vi "Posture Rotation.vi"(10 "Rotation X,Y,Z":cluster{"X":dbl, "Y":dbl, "Z":dbl}) -> (0 "angles":cluster{"roll":dbl, "pitch":dbl, "yaw":dbl}, 1 "Rotation Vector":dbl[](array[numeric]), 2 "Rotation Angle":dbl, 3 "data out":T1)   [LabVIEW 2021]
doc: "This VI calculates the Rotation Angle and Rotation\nVector between gravity acceleration in myRIO and \ngraivty const."
uses:
  ROVdataOut.ctl
panel:
  # "This VI calculates the Rotation Angle and Rotation\nVector between gravity acceleration in myRIO and \ngraivty const."
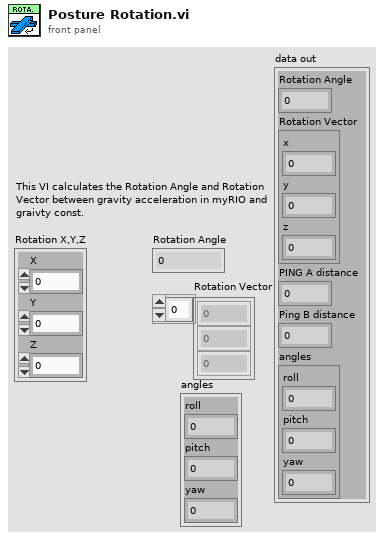
[diagram p1: front panel]
types:
  T1 = typedef "ROVdataOut.ctl" = cluster{"Rotation Angle":dbl, "Rotation Vector":cluster{"x":dbl, "y":dbl, "z":dbl}, "PING A distance":dbl, "Ping B distance":dbl, "angles":cluster{"roll":dbl, "pitch":dbl, "yaw":dbl}}
  T2 = typedef "NI_Matrix.lvlib/RealMatrix.ctl" = dbl[][]
  T3 = cluster{"Numeric":dbl, "Numeric":dbl, "Numeric":dbl}
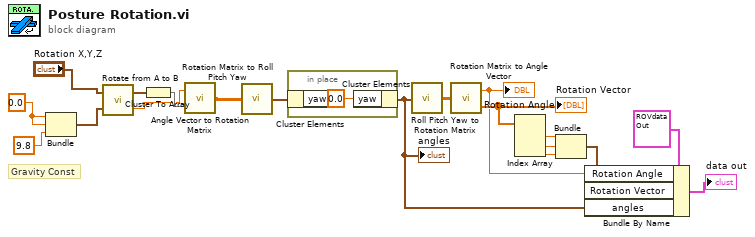
[diagram p0: block diagram]
diagram:
  w19 = 0.0
  # "Gravity Const"
  n1 = Bundle(w19, w19, 9.8) -> (w10:cluster{dbl, dbl, dbl})  [unwired: 1 in]
  n2 = call "Rotate from A to B.vi"("Vector B"=w10, "Vector A"="Rotation X,Y,Z") -> ("Rotation.Angle"=w12:dbl, "Rotation.Axis"=w13:cluster{"X":sgl, "Y":sgl, "Z":sgl})
  n3 = Cluster To Array(cluster=w13) -> (array=w14:sgl[])
  n4 = call "Angle Vector to Rotation Matrix.vi"("vector"=w14, "angle"=w12) -> ("rotation matrix"=w15:dbl[][])
  n5 = call "Rotation Matrix to Roll Pitch Yaw.vi"("rotation matrix"=w15) -> ("angles"=w16:cluster{"roll":dbl, "pitch":dbl, "yaw":dbl})
  n6 = in-place {
    n7 = in-place-cluster #1(w16) -> ()  [unwired: 1 out]
    n8 = in-place-cluster #1("yaw"=0.0) -> (w1:cluster{"roll":dbl, "pitch":dbl, "yaw":dbl})
  }
  "angles" <- w1
  n9 = call "Roll Pitch Yaw to Rotation Matrix.vi"("angles"=w1) -> ("rotation matrix"=w17:T2)
  n10 = call "Rotation Matrix to Angle Vector.vi"("rotation matrix"=w17) -> ("angle"=w4:dbl, "vector"=w9:dbl[])
  "Rotation Angle" <- w4
  "Rotation Vector" <- w9
  n11 = Index Array(array=w9) -> (element #1=w8:dbl, element #2=w7:dbl, element #3=w6:dbl)  [unwired: 3 in]
  n12 = Bundle("Numeric"=w8, "Numeric"=w7, "Numeric"=w6) -> (w5:T3)  [unwired: 1 in]
  n13 = Bundle By Name(cluster=T1 {"Rotation Angle"=0.0, "Rotation Vector"={"x"=0.0, "y"=0.0, "z"=0.0}, "PING A distance"=0.0, "Ping B distance"=0.0, "angles"={"roll"=0.0, "pitch"=0.0, "yaw"=0.0}} ("data out"), "Rotation Angle"=w4, "Rotation Vector"=w5, "angles"=w1) -> (→"data out":T1)
